vi "Test strain logger.vi"() -> ()   [LabVIEW 2024]
uses:
  Strain Logger.lvclass
  D:/GitHub/LabActor/Worker/Worker Actor/Worker Actor.lvclass
  NHMFL_Core/Libraries/Instruments/Results/File Path Result/File Path Result.lvclass
  D:/GitHub/NHMFL_Core/Libraries/Instruments/Results/Acquired Result/Acquired Result.lvclass
panel:
  out "error out":errorcluster
  out "Strain Logger out":refnum<class "Strain Logger.lvclass">
  in  "File Path":path
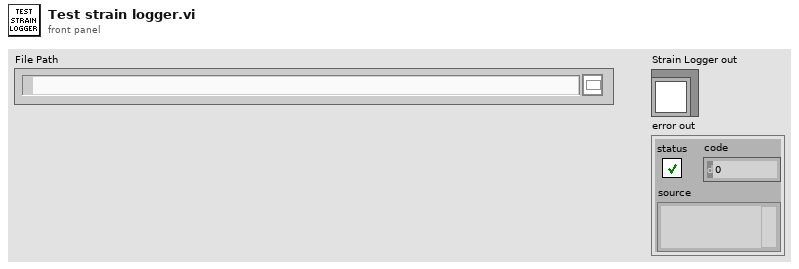
[diagram p1: front panel]
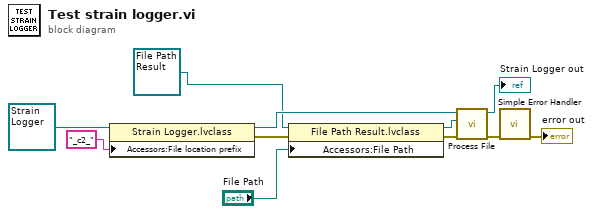
[diagram p0: block diagram]
diagram:
  n1 = property class="Strain Logger.lvclass"(reference=refnum<class "Strain Logger.lvclass"> refnum ("Strain Logger.lvclass"), "Accessors:File location prefix"="_c2_" ("File location prefix")) -> (reference out=w7:refnum<class "Strain Logger.lvclass">, error out=w8:errorcluster)  [unwired: 1 in]
  n2 = property class="File Path Result.lvclass"(reference=refnum<class "File Path Result.lvclass"> refnum ("File Path Result.lvclass"), error in=w8, "Accessors:File Path"="File Path") -> (reference out=w5:refnum<class "File Path Result.lvclass">, error out=w6:errorcluster)
  n3 = call-dynamic "Process File.vi"("error in (no error)"=w6, "Result in"=w5, "Strain Logger in"=w7) -> ("error out"=w3:errorcluster, "Strain Logger out"=→"Strain Logger out":refnum<class "Strain Logger.lvclass">)  [unwired: 6 in, 1 out]
  n4 = call <vilib>:"Simple Error Handler.vi"("error in (no error)"=w3) -> ("error out"=→"error out":errorcluster)  [unwired: 4 in, 4 out]
